vi "Get Test Data.vi"(8 "error in (no error)":errorcluster, 11 "Session Handle in":T4) -> (0 "error out":errorcluster, 2 "Test Data":T1[](array[typedef]), 3 "Session Handle out":T4)   [LabVIEW 2018, in "TestDataMgr.lvclass"]
uses:
  TestDataMgr.lvclass
  Typedefs/Session Handle.ctl
  Typedefs/Test Data All.ctl
  Typedefs/Test Limits.ctl
  Typedefs/Test Raw Data.ctl
  TestDataMgr.lvclass/TestDataMgr.ctl
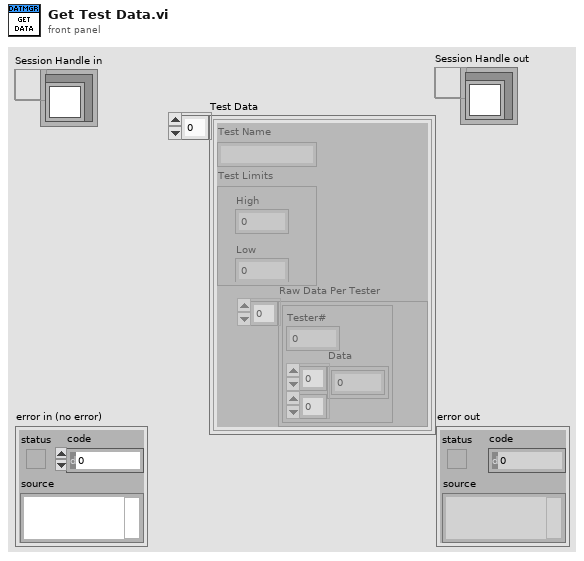
[diagram p1: front panel]
types:
  T1 = typedef "TestDataMgr.lvclass/Test Data All.ctl" = cluster{"Test Name":string, "Test Limits":T2, "Raw Data Per Tester":T3[]}
  T2 = typedef "TestDataMgr.lvclass/Test Limits.ctl" = cluster{"High":dbl, "Low":dbl}
  T3 = typedef "TestDataMgr.lvclass/Test Raw Data.ctl" = cluster{"Data":dbl[][], "Tester#":u8}
  T4 = typedef "TestDataMgr.lvclass/Session Handle.ctl" = refnum<data-value>
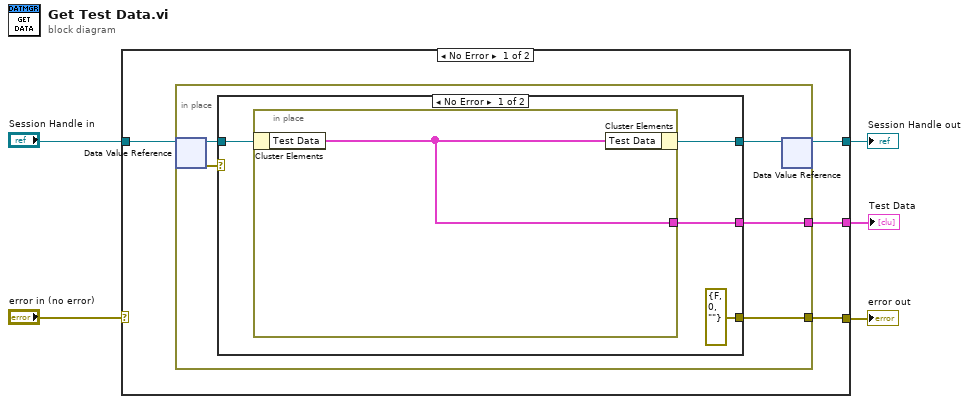
[diagram p0: block diagram]
diagram:
  n1 = case shown="No Error" "error in (no error)" {
    selector: "error in (no error)" -> [_ w23]
    tunnel: [w7 w23] -> w4
    tunnel: [w8 w22] -> w2
    tunnel: "Session Handle in" -> [w9 w22]
    tunnel: [w6 _] -> w1
    frame No Error {
      n2 = in-place {
        in-place-border: [w14] -> w7
        in-place-border: [w10] -> w6
        n3 = in-place-dvr #1(w9) -> (w12:refnum<class "TestDataMgr.lvclass">, w13:errorcluster)
        n4 = case shown="No Error" w13 {
          selector: w13 -> [_ w21]
          tunnel: [errorcluster {"status"=FALSE, "code"=0, "source"=""} ("error IO") w21] -> w14
          tunnel: w12 -> [w18 w20]
          tunnel: [w16 w20] -> w11
          tunnel: [w15 _] -> w10
          frame No Error {
            n5 = in-place {
              in-place-border: [w19] -> w15
              n6 = in-place-cluster #2(w18) -> ("Test Data"=w19:T1[])
              n7 = in-place-cluster #2("Test Data"=w19) -> (w16:refnum<class "TestDataMgr.lvclass">)
            }
          }
          frame Error {
          }
        }
        n8 = in-place-dvr #1(w11) -> (w8:T4)  [unwired: 1 out]
      }
    }
    frame Error {
    }
  }
  "error out" <- w4
  "Session Handle out" <- w2
  "Test Data" <- w1
